vi "encoderControlledHolonomicDrive.vi"(0 "RobotDriveDevRef":T1={"DevStatus"={"status"=FALSE, "code"=0, "source"=""}, "Motors[]"=[], "Square Inputs"=FALSE, "Max Output"=1.0}, 5 "X":dbl, 7 "Y":dbl, 9 "Rotation":dbl, 11 "error in (no error)":errorcluster, 12 "Encoder Readings":dbl[](array[numeric])) -> (4 "RobotDriveDevRef":T1={"DevStatus"={"status"=FALSE, "code"=0, "source"=""}, "Motors[]"=[], "Square Inputs"=FALSE, "Max Output"=1.0}, 8 "Motor Values":dbl[](array[numeric]), 15 "error out":errorcluster)   [LabVIEW 2014]
uses:
  <vilib>/Rock Robotics/WPI/RobotDrive/WPI_RobotDriveDevRef.ctl
  <vilib>/Rock Robotics/WPI/MotorControl/WPI_MotorControlDeviceRef.ctl
  <vilib>/Rock Robotics/WPI/MotorControl/WPI_MotorControlType.ctl
  <vilib>/Rock Robotics/SystemInterfaces/Typedef/FPGA_TypedefDigitalModule.ctl
  <vilib>/Rock Robotics/SystemInterfaces/DIO/FPGA_DIOPWMChannel.ctl
  <vilib>/Rock Robotics/WPI/PWM/WPI_PWMDeadband.ctl
  <vilib>/Rock Robotics/WPI/CAN/Jaguar/SubVIs/WPI_CANJaguar_ControlMode.ctl
  <vilib>/Rock Robotics/WPI/CAN/TalonSRX/WPI_CANTalonSRX_APIControlMode.ctl
  <vilib>/Rock Robotics/WPI/PWM/WPI_PWMTransform_ConPane.ctl
  <vilib>/Rock Robotics/SystemInterfaces/NetworkCommunication/NetComm_UsageReport_ResourceType.ctl
  <vilib>/Rock Robotics/WPI/RobotDrive/WPI_RobotDriveMotorSelectorEnum.ctl
  <vilib>/Rock Robotics/WPI/RobotDrive/WPI_RobotDriveSafetyCheck.vi
panel:
  in  "Proportional Constant":dbl
  in  "Gyro Angle":dbl
  # "**********************************************"
  # "Make sure this value is 0.046 every time"
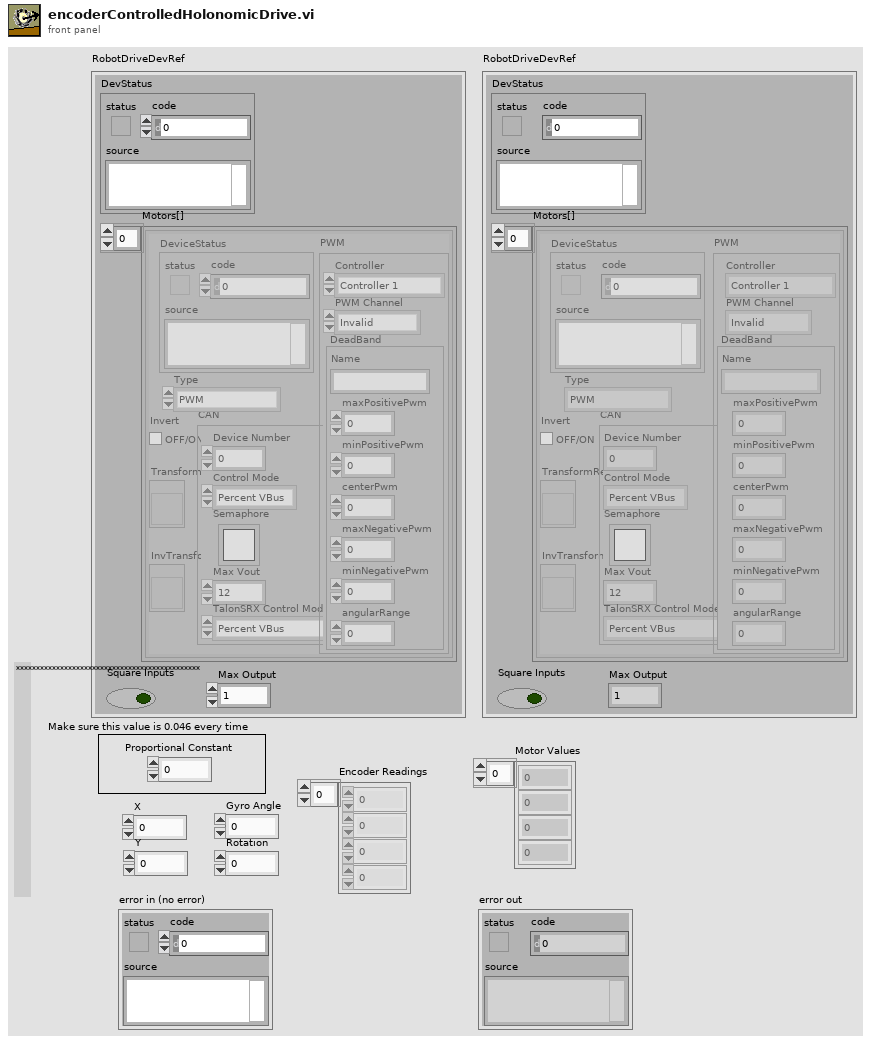
[diagram p1: front panel]
types:
  T1 = typedef "WPI_RobotDriveDevRef.ctl" = cluster{"DevStatus":errorcluster, "Motors[]":T2[], "Square Inputs":bool, "Max Output":dbl}
  T2 = typedef "WPI_MotorControlDeviceRef.ctl" = cluster{"DeviceStatus":errorcluster, "Type":T3, "PWM":cluster{"Controller":T4, "PWM Channel":T5, "DeadBand":T6}, "CAN":cluster{"Device Number":u8, "Control Mode":T7, "Semaphore":T8, "Max Vout":dbl, "TalonSRX Control Mode":T9}, "Invert":bool, "TransformRef":T10, "InvTransformRef":T10}
  T3 = typedef "WPI_MotorControlType.ctl" = enum16{"PWM", "CAN", "CANTalonSRX"}
  T4 = typedef "FPGA_TypedefDigitalModule.ctl" = enum16{"Controller 1"}
  T5 = typedef "FPGA_DIOPWMChannel.ctl" = enum8{"PWM 0", "PWM 1", "PWM 2", "PWM 3", "PWM 4", "PWM 5", "PWM 6", "PWM 7", "PWM 8", "PWM 9", "PWM MXP 0", "PWM MXP 1", "PWM MXP 2", "PWM MXP 3", "PWM MXP 4", "PWM MXP 5", "PWM MXP 6", "PWM MXP 7", "PWM MXP 8", "PWM MXP 9", "Invalid"}
  T6 = typedef "WPI_PWMDeadband.ctl" = cluster{"Name":string, "maxPositivePwm":i32, "minPositivePwm":i32, "centerPwm":i32, "maxNegativePwm":i32, "minNegativePwm":i32, "angularRange":u16}
  T7 = typedef "WPI_CANJaguar_ControlMode.ctl" = enum8{"Percent VBus", "Current", "Speed", "Position", "Voltage"}
  T8 = typedef "Semaphore RefNum" = refnum<k1>
  T9 = typedef "WPI_CANTalonSRX_APIControlMode.ctl" = enum8{"Percent VBus", "Speed", "Position", "Slave", "Unchanged / Invalid"}
  T10 = typedef "WPI_PWMTransform_ConPane.ctl" = refnum<vi>
  T11 = typedef "NetComm_UsageReport_ResourceType.ctl" = enum8{"Controller", "Module", "Language", "CANPlugin", "Accelerometer", "ADXL345", "AnalogChannel", "AnalogTrigger", "AnalogTriggerOutput", "CANJaguar", "Compressor", "Counter", "Dashboard", "DigitalInput", "DigitalOutput", "DriverStationCIO", "DriverStationEIO", "DriverStationLCD", "Encoder", "GearTooth", "Gyro", "I2C", "Framework", "Jaguar", "Joystick", "Kinect", "KinectStick", "PIDController", "Preferences", "PWM", "Relay", "RobotDrive", "SerialPort", "Servo", "Solenoid", "SPI", "Task", "Ultrasonic", "Victor", "Button", "Command", "AxisCamera", "PCVideoServer", "SmartDashboard", "Talon", "HiTechnicColorSensor", "HiTechnicAccel", "HiTechnicCompass", "SRF08", "AnalogOutput", "Victor SP", "Talon SRX", "CAN Talon SRX"}
  T12 = typedef "WPI_RobotDriveMotorSelectorEnum.ctl" = enum16{"Rear Left Motor", "Rear Right Motor", "Front Left Motor", "Front Right Motor"}
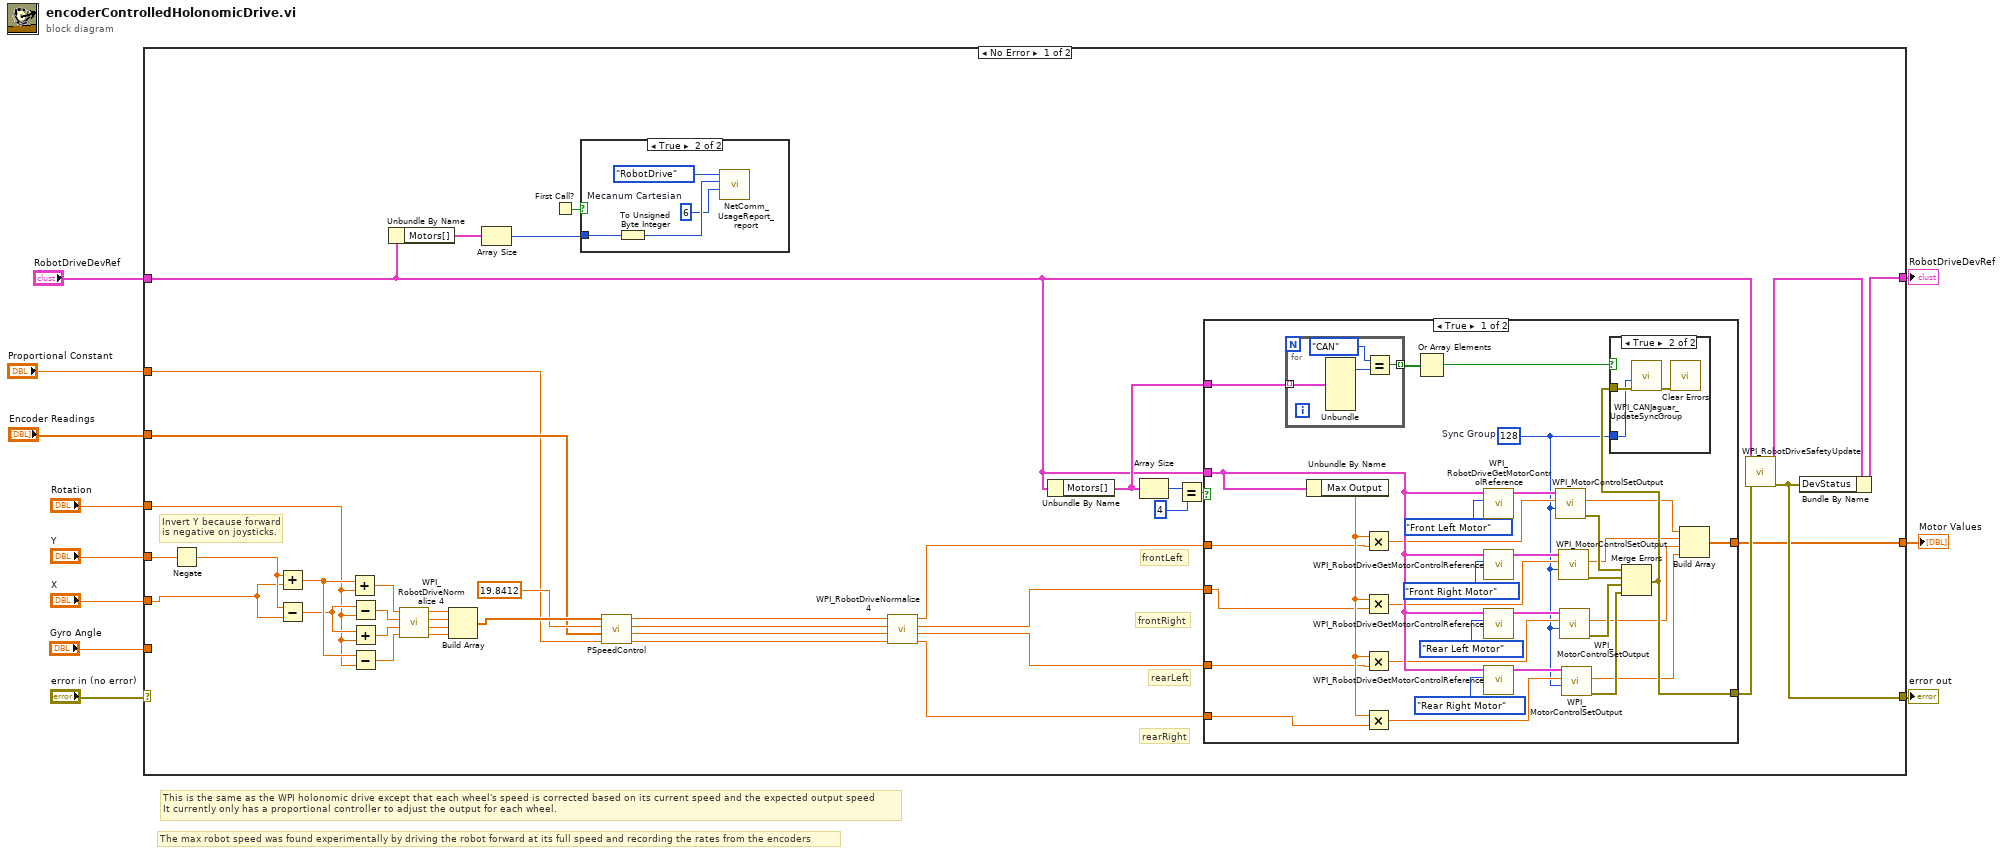
[diagram p0: block diagram]
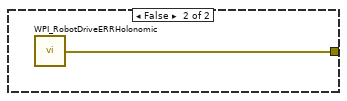
[diagram p4: hidden frame]
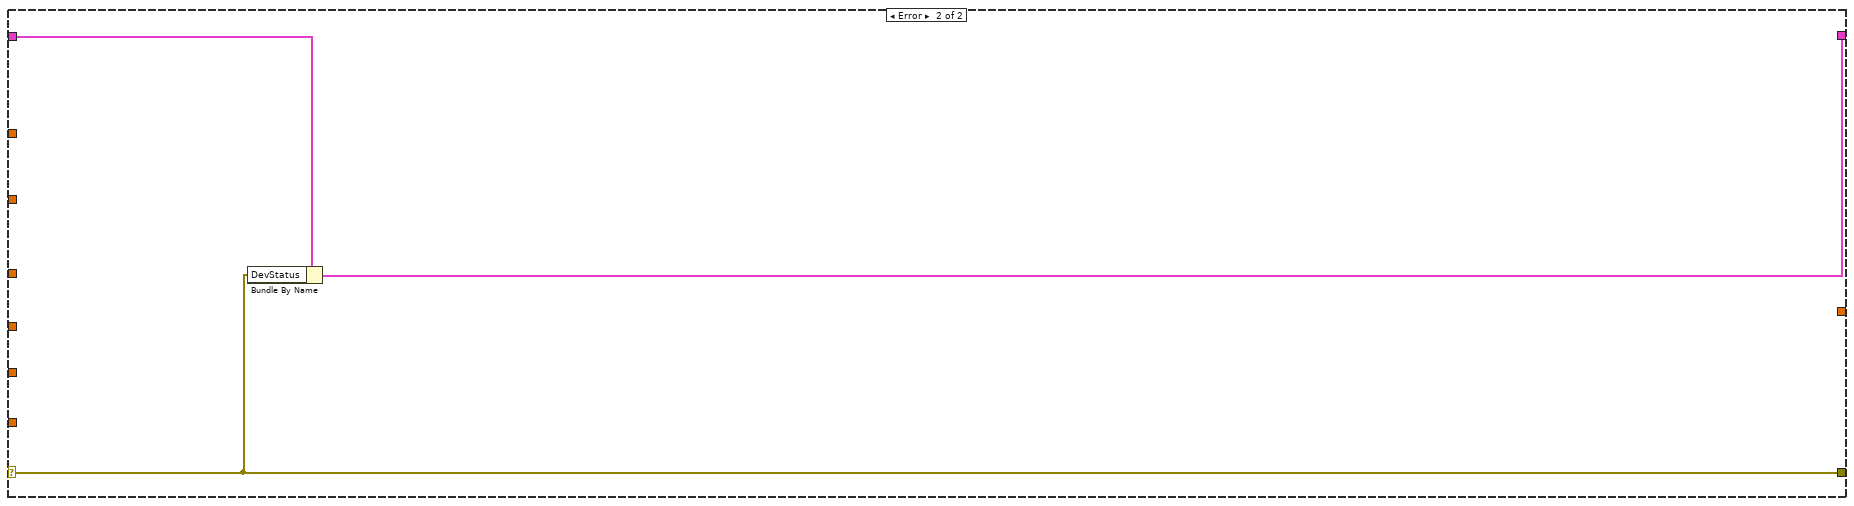
[diagram p5: hidden frame]
diagram:
  # "The max robot speed was found experimentally by driving the robot forward at its full speed and recording the rates from the encoders"
  # "This is the same as the WPI holonomic drive except that each wheel's speed is corrected based on its current speed and the expected output speed\nIt currently only has a proportional controller to adjust the output for each wheel."
  n1 = case shown="No Error" "error in (no error)" {
    selector: "error in (no error)" -> [_ w95]
    tunnel: "Y" -> [w39 _]
    tunnel: "X" -> [w28 _]
    tunnel: "RobotDriveDevRef" -> [w31 w97]
    tunnel: [w47 w96] -> w7
    tunnel: [w36 w95] -> w6
    tunnel: "Rotation" -> [w40 _]
    tunnel: "Gyro Angle" -> [_ _]
    tunnel: [w30 _] -> w3
    tunnel: "Proportional Constant" -> [w15 _]
    tunnel: "Encoder Readings" -> [w16 _]
    frame No Error {
      # "Invert Y because forward is negative on joysticks."
      # "rearLeft"
      # "frontRight"
      # "rearRight"
      # "frontLeft"
      n2 = Negate(x=w39) -> (-x=w29:dbl)
      n3 = Add(x=w29, y=w28) -> (x+y=w45:dbl)
      n4 = Subtract(x=w29, y=w28) -> (x-y=w43:dbl)
      n5 = Add(x=w45, y=w40) -> (x+y=w41:dbl)
      n6 = Subtract(x=w43, y=w40) -> (x-y=w42:dbl)
      n7 = Add(x=w43, y=w40) -> (x+y=w44:dbl)
      n8 = Subtract(x=w45, y=w40) -> (x-y=w46:dbl)
      n9 = Unbundle By Name(w31) -> ("Motors[]"=w33:T2[])
      n10 = call <vilib>:"WPI_RobotDriveNormalize 4.vi"("D"=w46, "C"=w44, "B"=w42, "A"=w41) -> ("D'"=w19:dbl, "C'"=w20:dbl, "B'"=w21:dbl, "A'"=w22:dbl)
      n11 = Build Array(w22, w21, w20, w19) -> (w18:dbl[])
      n12 = Array Size(array=w33) -> (size(s)=w32:i32)
      n13 = First Call?() -> (First Call?: T/F=w34:bool)
      n14 = case shown="True" w34 {
        tunnel: w32 -> [_ w53]
        frame False {
        }
        frame True {
          w51 = u8 6  # Mecanum Cartesian
          n15 = To Unsigned Byte Integer(number=w53) -> (unsigned 8bit integer=w52:u8)
          n16 = call <vilib>:"NetComm_UsageReport_report.vi"("Context"=w51, "Instance Number"=w52, "Resource Type"=NetComm_UsageReport_ResourceType."RobotDrive") -> ()  [unwired: 9 in]
        }
      }
      n17 = call "PSpeedControl.vi"("Proportional Constant"=w15, "Current Encoder Rates"=w16, "Robot Max Rate"=19.8412 ("Maximum Rate"), "Targets"=w18) -> ("Motor Output 4"=w12:dbl, "Motor Output 3"=w13:dbl, "Motor Output 2"=w14:dbl, "Motor Output 1"=w23:dbl)  [unwired: 4 in]
      n18 = call <vilib>:"WPI_RobotDriveNormalize 4.vi"("D"=w12, "C"=w13, "B"=w14, "A"=w23) -> ("D'"=w24:dbl, "C'"=w25:dbl, "B'"=w26:dbl, "A'"=w27:dbl)
      n19 = Unbundle By Name(w31) -> ("Motors[]"=w35:T2[])
      n20 = Array Size(array=w35) -> (size(s)=w50:i32)
      n21 = Equal?(x=w50, y=4) -> (x = y?=w48:bool)
      n22 = case shown="True" w48 {
        tunnel: w31 -> [w78 _]
        tunnel: [w65 w94] -> w38
        tunnel: w35 -> [w66 _]
        tunnel: [w62 _] -> w30
        tunnel: w27 -> [w58 _]
        tunnel: w26 -> [w57 _]
        tunnel: w25 -> [w56 _]
        tunnel: w24 -> [w55 _]
        frame True {
          w64 = u8 128  # Sync Group
          n23 = for {
            tunnel: w66 -> [w90] mode=indexing
            tunnel: [w87] -> w67 mode=indexing
            n24 = Unbundle(w90) -> ("Type"=w89:T3)  [unwired: 6 out]
            n25 = Equal?(x=enum16{"PWM", "CAN"}."CAN" ("Type"), y=w89) -> (x = y?=w87:bool)
          }
          n26 = Unbundle By Name(w78) -> ("Max Output"=w73:dbl)
          n27 = Multiply(x=w73, y=w58) -> (x*y=w77:dbl)
          n28 = Multiply(x=w73, y=w57) -> (x*y=w76:dbl)
          n29 = Multiply(x=w73, y=w56) -> (x*y=w75:dbl)
          n30 = Multiply(x=w73, y=w55) -> (x*y=w74:dbl)
          n31 = Or Array Elements(Boolean array=w67) -> (logical OR=w68:bool)
          n32 = call <vilib>:"WPI_RobotDriveGetMotorControlReference.vi"("MotorIndex"=WPI_RobotDriveMotorSelectorEnum."Front Left Motor", "RobotDriveDevRef"=w78) -> ("MotorControlDeviceRef"=w86:T2)  [unwired: 9 out]
          n33 = call <vilib>:"WPI_RobotDriveGetMotorControlReference.vi"("MotorIndex"=WPI_RobotDriveMotorSelectorEnum."Front Right Motor", "RobotDriveDevRef"=w78) -> ("MotorControlDeviceRef"=w84:T2)  [unwired: 9 out]
          n34 = call <vilib>:"WPI_RobotDriveGetMotorControlReference.vi"("MotorIndex"=WPI_RobotDriveMotorSelectorEnum."Rear Left Motor", "RobotDriveDevRef"=w78) -> ("MotorControlDeviceRef"=w85:T2)  [unwired: 9 out]
          n35 = call <vilib>:"WPI_RobotDriveGetMotorControlReference.vi"("MotorIndex"=WPI_RobotDriveMotorSelectorEnum."Rear Right Motor", "RobotDriveDevRef"=w78) -> ("MotorControlDeviceRef"=w83:T2)  [unwired: 9 out]
          n36 = call <vilib>:"WPI_MotorControlSetOutput.vi"("Sync Group / Parameter Slot"=w64, "Output"=w77, "MotorControlDevRef"=w86) -> ("error out"=w69:errorcluster, "Motor Output"=w63:dbl)  [unwired: 2 in, 5 out]
          n37 = call <vilib>:"WPI_MotorControlSetOutput.vi"("Sync Group / Parameter Slot"=w64, "Output"=w76, "MotorControlDevRef"=w84) -> ("error out"=w70:errorcluster, "Motor Output"=w61:dbl)  [unwired: 2 in, 5 out]
          n38 = call <vilib>:"WPI_MotorControlSetOutput.vi"("Sync Group / Parameter Slot"=w64, "Output"=w75, "MotorControlDevRef"=w85) -> ("error out"=w71:errorcluster, "Motor Output"=w60:dbl)  [unwired: 2 in, 5 out]
          n39 = call <vilib>:"WPI_MotorControlSetOutput.vi"("Sync Group / Parameter Slot"=w64, "Output"=w74, "MotorControlDevRef"=w83) -> ("error out"=w72:errorcluster, "Motor Output"=w59:dbl)  [unwired: 2 in, 5 out]
          n40 = Merge Errors(w69, w70, w71, w72) -> (w65:errorcluster)
          n41 = case shown="True" w68 {
            tunnel: w65 -> [_ w92]
            tunnel: w64 -> [_ w91]
            frame False {
            }
            frame True {
              n42 = call <vilib>:"WPI_CANJaguar_UpdateSyncGroup.vi"("error in (no error)"=w92, "Sync Group"=w91) -> ("error out"=w93:errorcluster)  [unwired: 9 out]
              n43 = call <vilib>:"Clear Errors.vi"("error in (no error)"=w93) -> ()  [unwired: 1 in, 6 out]
            }
          }
          n44 = Build Array(w63, w61, w60, w59) -> (w62:dbl[])
        }
        frame False {
          n45 = call <vilib>:"WPI_RobotDriveERRHolonomic.vi"() -> ("error out"=w94:errorcluster)
        }
      }
      n46 = call <vilib>:"WPI_RobotDriveSafetyUpdate.vi"("error in (no error)"=w38, "RobotDriveDevRef"=w31) -> ("error out"=w36:errorcluster, "RobotDriveDevRef"=w37:T1)  [unwired: 8 out]
      n47 = Bundle By Name(cluster=w37, "DevStatus"=w36) -> (w47:T1)
    }
    frame Error {
      n48 = Bundle By Name(cluster=w97, "DevStatus"=w95) -> (w96:T1)
    }
  }
  "error out" <- w6
  "RobotDriveDevRef" <- w7
  "Motor Values" <- w3
